vi "Meas Proc QWTB Write Algorithm Processing Header.vi"(7 "processing setup":T1={"mode"=enum."Raw", "call after avgs?"=FALSE, "calculate?"=FALSE, "raw mode"={"command"="", "result mode"=enum."Display console output (only Octave)", "res variable"=""}, "QWTB"={"QWTB path"=path "", "alg filter path"="", "alg ids"=[], "alg parameters"=[], "parsed parameters"=[], "selected alg id"="", "selected unc mode"=enum."None", "qwtb mcc"=100, "qwtb timeout"=90, "qwtb covg"=95.0, "qwtb ofs"=0, "qwtb lim data"=0, "multicore"={"jobs folder"=path "", "cores"=0, "max jobs"=0, "mode"=enum."Singlecore"}, "unc once?"=FALSE}}, 8 "error in":errorcluster, 11 "sequence item":T10) -> (0 "error out":errorcluster)   [LabVIEW 2018]
doc: "This VI will write QWTB calculation data into the info header file in the measurement root folder."
uses:
  Meas Sequence Item.ctl
  Meas Sampling Configuration.ctl
  adc/ADC Trig Config.ctl
  adc/ADC Trig Mode Source.ctl
  adc/ADC Trig Coupling.ctl
  adc/ADC Trig Slope.ctl
  Meas Proc QWTB Algorithm Parameter Data.ctl
  Meas Process Config.ctl
  Meas Process Mode.ctl
  Meas Process Raw Config.ctl
  Meas Process Raw Result Mode.ctl
  Meas Proc QWTB Setup.ctl
  Meas Proc QWTB Uncertainty Mode.ctl
  Meas Proc QWTB Multicore Setup.ctl
  Meas Proc QWTB Multicore Type.ctl
  octave/infolib.lvlibp
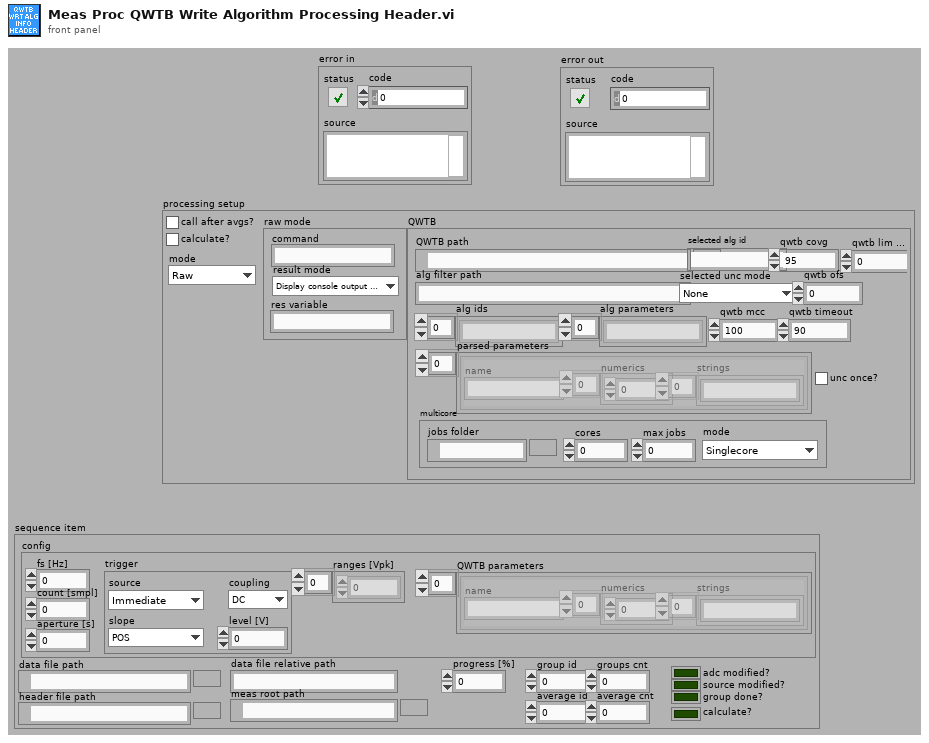
[diagram p1: front panel]
types:
  T1 = typedef "Meas Process Config.ctl" = cluster{"mode":T2, "call after avgs?":bool, "calculate?":bool, "raw mode":T3, "QWTB":T5}
  T2 = typedef "Meas Process Mode.ctl" = enum16{"Raw", "QWTB"}
  T3 = typedef "Meas Process Raw Config.ctl" = cluster{"command":string, "result mode":T4, "res variable":string}
  T4 = typedef "Meas Process Raw Result Mode.ctl" = enum16{"Display console output (only Octave)", "Display string variable", "Display result file %respath%"}
  T5 = typedef "Meas Proc QWTB Setup.ctl" = cluster{"QWTB path":path, "alg filter path":string, "alg ids":string[], "alg parameters":string[], "parsed parameters":T6[], "selected alg id":string, "selected unc mode":T7, "qwtb mcc":i32, "qwtb timeout":i32, "qwtb covg":dbl, "qwtb ofs":i64, "qwtb lim data":i64, "multicore":T8, "unc once?":bool}
  T6 = typedef "Meas Proc QWTB Algorithm Parameter Data.ctl" = cluster{"name":string, "numerics":dbl[], "strings":string[]}
  T7 = typedef "Meas Proc QWTB Uncertainty Mode.ctl" = enum16{"None", "GUF", "Monte Carlo"}
  T8 = typedef "Meas Proc QWTB Multicore Setup.ctl" = cluster{"jobs folder":path, "cores":i32, "max jobs":i32, "mode":T9}
  T9 = typedef "Meas Proc QWTB Multicore Type.ctl" = enum16{"Singlecore", "Multicore", "Multistation"}
  T10 = typedef "Meas Sequence Item.ctl" = cluster{"config":T11, "data file path":path, "header file path":path, "group id":i32, "average id":i32, "group done?":bool, "adc modified?":bool, "source modified?":bool, "progress [%]":dbl, "groups cnt":i32, "average cnt":i32, "data file relative path":string, "meas root path":path, "calculate?":bool}
  T11 = typedef "Meas Sampling Configuration.ctl" = cluster{"fs [Hz]":dbl, "count [smpl]":i64, "aperture [s]":dbl, "trigger":T12, "ranges [Vpk]":dbl[], "QWTB parameters":T6[]}
  T12 = typedef "ADC Trig Config.ctl" = cluster{"source":T13, "level [V]":dbl, "coupling":T14, "slope":T15}
  T13 = typedef "ADC Trig Mode Source.ctl" = enum16{"Immediate", "External", "Level"}
  T14 = typedef "ADC Trig Coupling.ctl" = enum16{"DC", "AC"}
  T15 = typedef "ADC Trig Slope.ctl" = enum16{"POS", "NEG"}
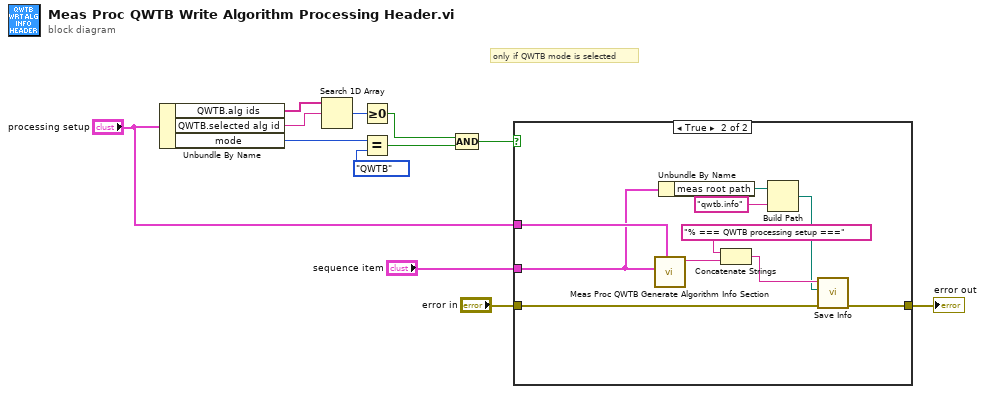
[diagram p0: block diagram]
diagram:
  # "only if QWTB mode is selected"
  n1 = Unbundle By Name("processing setup") -> ("QWTB.alg ids"=w3:string[], "QWTB.selected alg id"=w2:string, "mode"=w11:T2)
  n2 = Search 1D Array(1D array=w3, element=w2) -> (index of element=w1:i32)  [unwired: 1 in]
  n3 = Greater Or Equal To 0?(x=w1) -> (x >= 0?=w8:bool)
  n4 = Equal?(x=w11, y=Meas_Process_Mode."QWTB") -> (x = y?=w9:bool)
  n5 = Compound Arithmetic op=AND(w8, w9) -> (w7:bool)
  n6 = case shown="True" w7 {
    tunnel: "sequence item" -> [_ w19]
    tunnel: "processing setup" -> [_ w23]
    tunnel: "error in" -> [w13 w20]
    tunnel: [w13 w14] -> w4
    frame False {
    }
    frame True {
      n7 = call "Meas Proc QWTB Generate Algorithm Info Section.vi"("processing setup"=w23, "sequence item"=w19) -> ("new info data out"=w22:string)  [unwired: 8 in, 1 out]
      n8 = Unbundle By Name(w19) -> ("meas root path"=w18:path)
      n9 = Concatenate Strings("% === QWTB processing setup ===" ("string"), w22) -> (w21:string)
      n10 = Build Path(base path=w18, name or relative path="qwtb.info") -> (appended path=w16:path)
      n11 = call "Save Info.vi"("error in"=w20, "filename"=w16, "info data"=w21) -> ("error out"=w14:errorcluster)  [unwired: 8 in]
    }
  }
  "error out" <- w4
